vi "afslaan_deel2 (SubVI).vi"(7 "universele stop":bool, 8 "OK Button":bool, 11 "String":string) -> (3 "afslag gedaan":i32)   [LabVIEW 2019]
panel:
  out "rechtermotor : r":dbl=0.4
  out "linkermotor : r":dbl
  out "linkermotor : l":dbl=0.4
  out "rechtermotor : l":dbl
  out "rechtermotor : d":dbl=0.4
  out "linkermotor : d":dbl=0.4
  out "welke afslag is bezig":i32=1
  in  "stop":bool
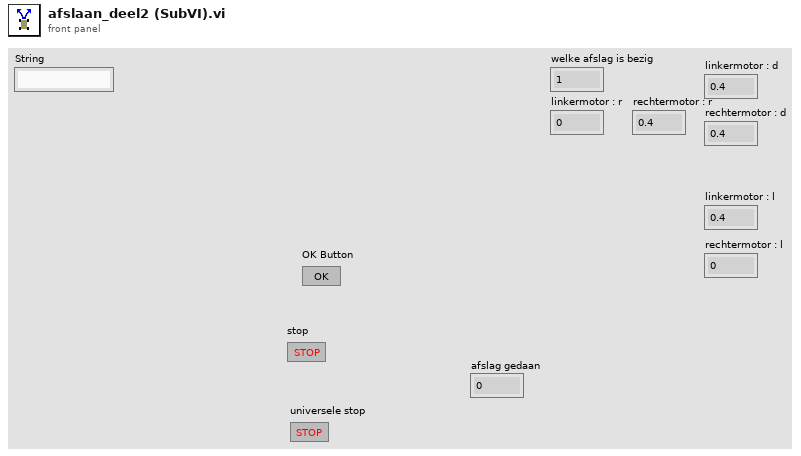
[diagram p1: front panel]
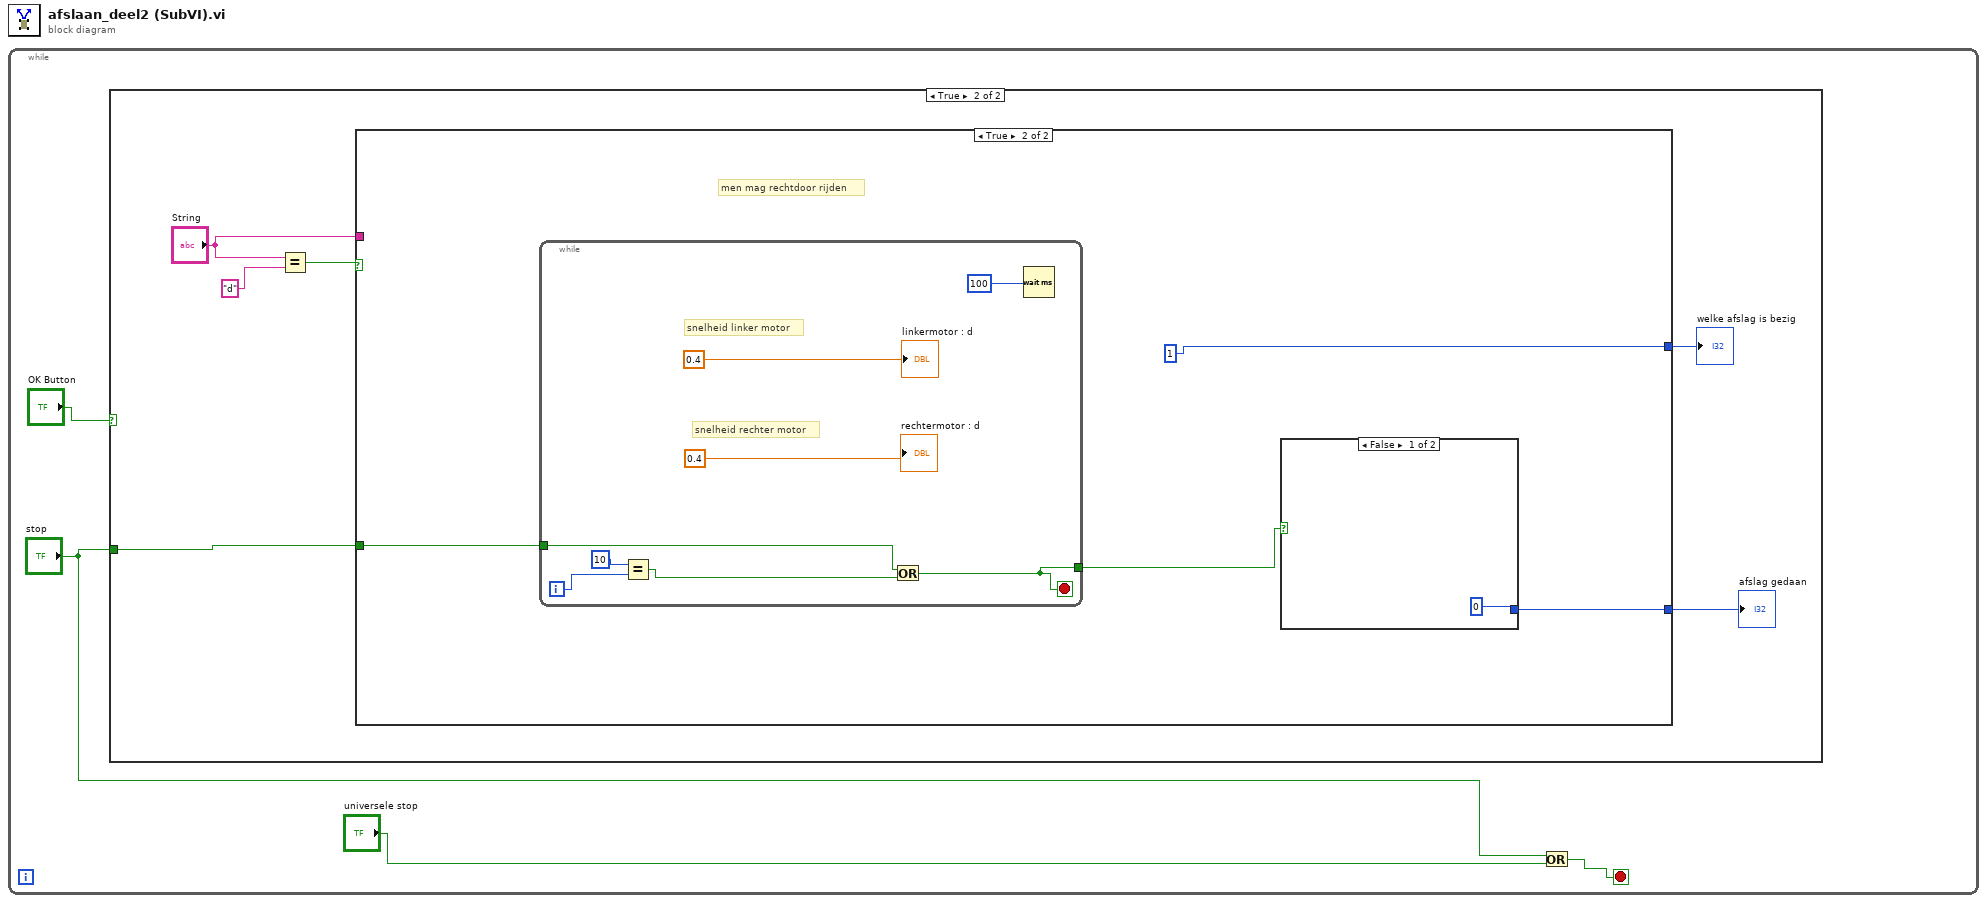
[diagram p0: block diagram]
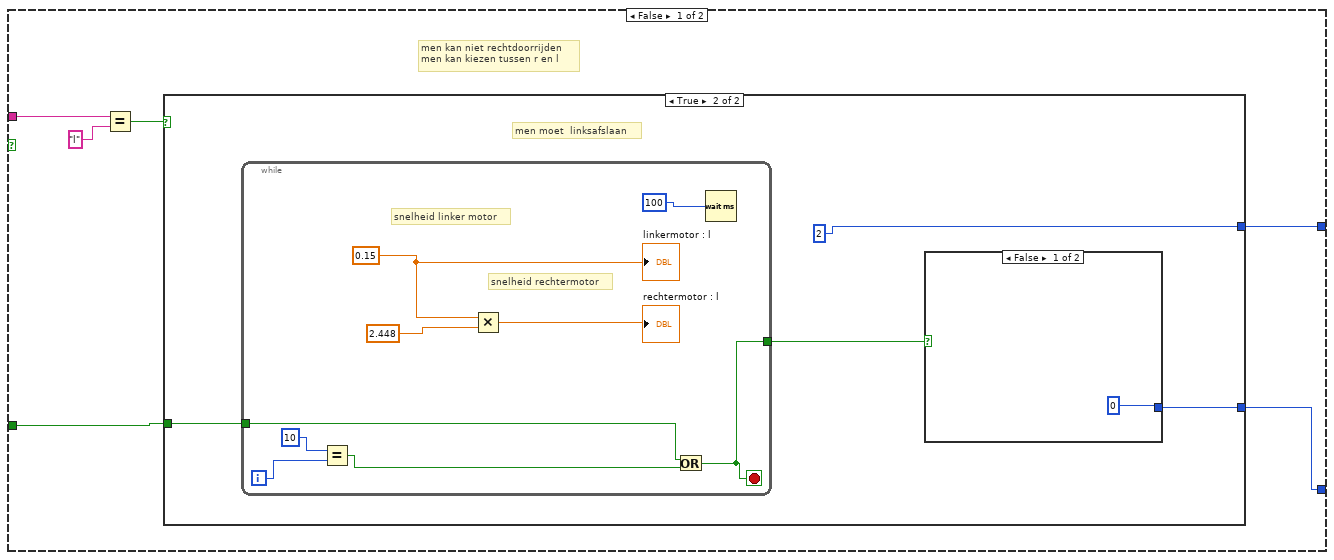
[diagram p3: hidden frame]
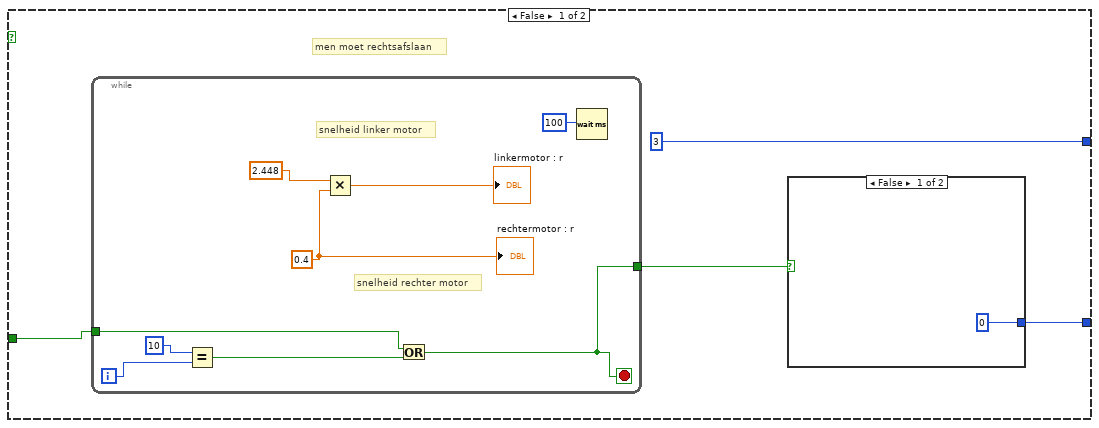
[diagram p4: hidden frame]
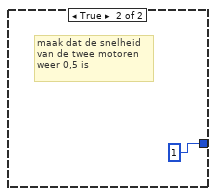
[diagram p5: hidden frame]
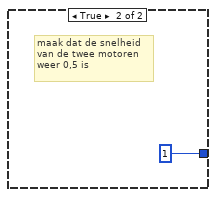
[diagram p6: hidden frame]
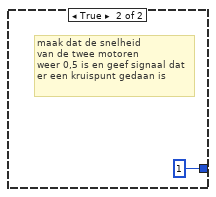
[diagram p7: hidden frame]
diagram:
  n1 = while {
    stop <- w4 stop-if-true
    n2 = case shown="True" "OK Button" {
      tunnel: "stop" -> [_ w6]
      frame False {
      }
      frame True {
        n3 = Equal?(x="String", y="d") -> (x = y?=w9:bool)
        n4 = case shown="True" w9 {
          tunnel: "String" -> [w14 _]
          tunnel: [w13 1] -> w7
          tunnel: w6 -> [w12 w49]
          tunnel: [w11 w47] -> w5
          frame False {
            # "men kan niet rechtdoorrijden \nmen kan kiezen tussen r en l"
            n5 = Equal?(x=w14, y="l") -> (x = y?=w16:bool)
            n6 = case shown="True" w16 {
              tunnel: [3 2] -> w13
              tunnel: w12 -> [w19 w34]
              tunnel: [w17 w32] -> w11
              frame False {
                # "men moet rechtsafslaan"
                n7 = while {
                  tunnel: w19 -> [w28]
                  tunnel: [w23] -> w18
                  i -> [w31]
                  stop <- w23 stop-if-true
                  w26 = 0.4
                  # "snelheid rechter motor"
                  # "snelheid linker motor"
                  n8 = Equal?(x=10, y=w31) -> (x = y?=w29:bool)
                  n9 = Multiply(x=2.448, y=w26) -> (x*y=→"linkermotor : r":dbl)
                  n10 = Or(x=w28, y=w29) -> (x .or. y?=w23:bool)
                  n11 = Wait (ms)(milliseconds to wait=100) -> ()  [unwired: 1 out]
                  "rechtermotor : r" <- w26
                }
                n12 = case shown="False" w18 {
                  tunnel: [0 1] -> w17
                  frame False {
                  }
                  frame True {
                    # "maak dat de snelheid \nvan de twee motoren\nweer 0,5 is"
                  }
                }
              }
              frame True {
                # "men moet  linksafslaan"
                n13 = while {
                  tunnel: w34 -> [w42]
                  tunnel: [w38] -> w33
                  i -> [w45]
                  stop <- w38 stop-if-true
                  w41 = 0.15
                  # "snelheid rechtermotor"
                  # "snelheid linker motor"
                  n14 = Equal?(x=10, y=w45) -> (x = y?=w43:bool)
                  n15 = Multiply(x=w41, y=2.448) -> (x*y=→"rechtermotor : l":dbl)
                  n16 = Or(x=w42, y=w43) -> (x .or. y?=w38:bool)
                  n17 = Wait (ms)(milliseconds to wait=100) -> ()  [unwired: 1 out]
                  "linkermotor : l" <- w41
                }
                n18 = case shown="False" w33 {
                  tunnel: [0 1] -> w32
                  frame False {
                  }
                  frame True {
                    # "maak dat de snelheid \nvan de twee motoren\nweer 0,5 is"
                  }
                }
              }
            }
          }
          frame True {
            # "men mag rechtdoor rijden"
            n19 = while {
              tunnel: w49 -> [w57]
              tunnel: [w53] -> w48
              i -> [w59]
              stop <- w53 stop-if-true
              # "snelheid rechter motor"
              # "snelheid linker motor"
              n20 = Equal?(x=10, y=w59) -> (x = y?=w58:bool)
              n21 = Or(x=w57, y=w58) -> (x .or. y?=w53:bool)
              n22 = Wait (ms)(milliseconds to wait=100) -> ()  [unwired: 1 out]
              "linkermotor : d" <- 0.4
              "rechtermotor : d" <- 0.4
            }
            n23 = case shown="False" w48 {
              tunnel: [0 1] -> w47
              frame False {
              }
              frame True {
                # "maak dat de snelheid \nvan de twee motoren\nweer 0,5 is en geef signaal dat\ner een kruispunt gedaan is"
              }
            }
          }
        }
        "welke afslag is bezig" <- w7
        "afslag gedaan" <- w5
      }
    }
    n24 = Or(x="stop", y="universele stop") -> (x .or. y?=w4:bool)
  }
